vi "Align with Shape.vi"(7 "Margin":cluster{"Horizontal":u32, "Vertical":u32}, 8 "error in (no error)":errorcluster, 9 "Alignment":T1(ring), 10 "Reference Shape":refnum<class "Shape.lvclass">, 11 "Shape in":refnum<class "Shape.lvclass">) -> (0 "error out":errorcluster, 3 "Shape out":refnum<class "Shape.lvclass">)   [LabVIEW 2015, in "LV Image Editor Framework.lvlib" / "Shape.lvclass"]
uses:
  Shape.lvclass
  Shape.lvclass/Shape.ctl
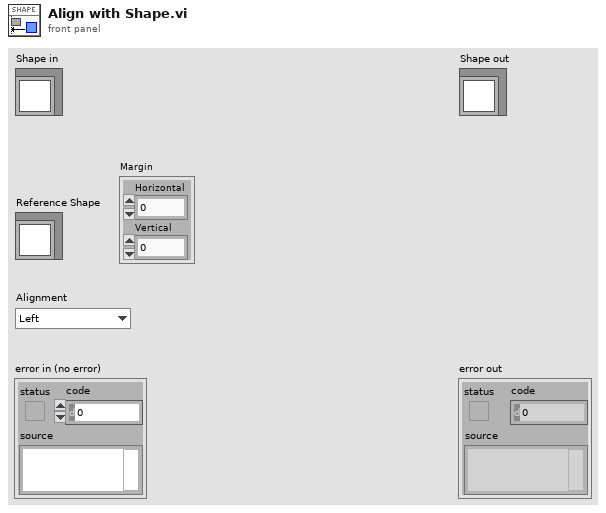
[diagram p1: front panel]
types:
  T1 = enum16{"Left", "Top", "Right", "Bottom", "Centered"}
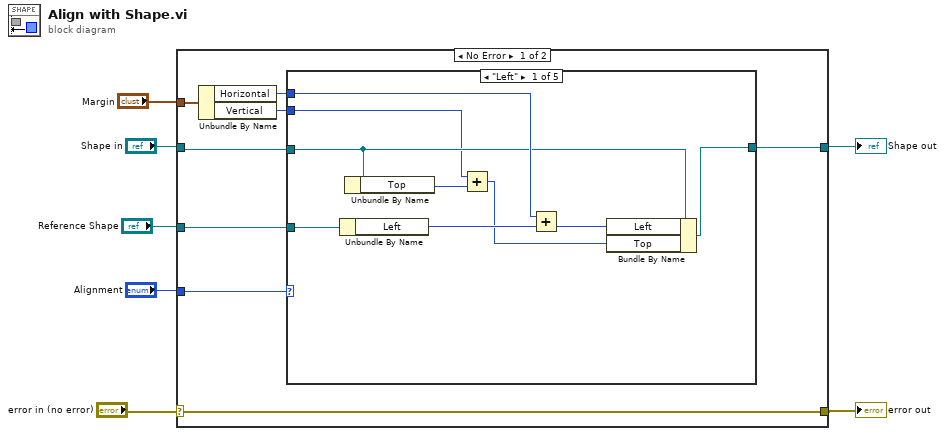
[diagram p0: block diagram]
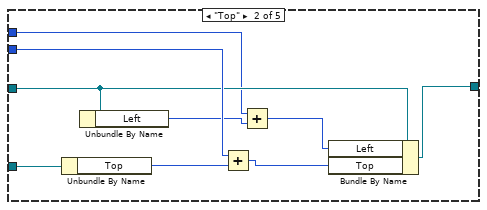
[diagram p2: hidden frame]
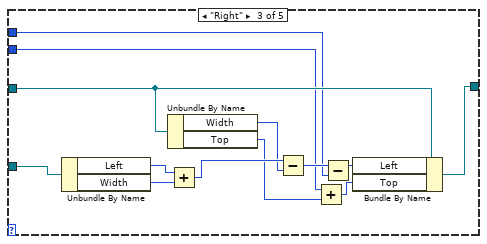
[diagram p3: hidden frame]
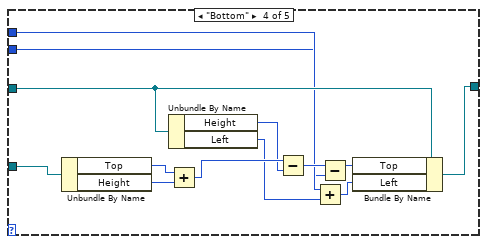
[diagram p4: hidden frame]
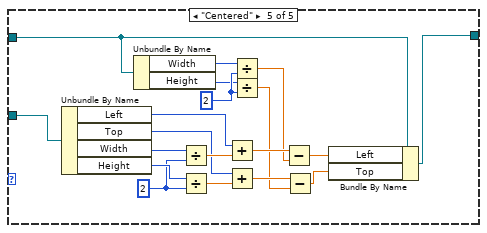
[diagram p5: hidden frame]
diagram:
  n1 = case shown="No Error" "error in (no error)" {
    selector: "error in (no error)" -> [w15 w80]
    tunnel: [w15 w80] -> w6
    tunnel: [w11 w79] -> w2
    tunnel: "Shape in" -> [w13 w79]
    tunnel: "Alignment" -> [w14 _]
    tunnel: "Reference Shape" -> [w12 _]
    tunnel: "Margin" -> [w10 _]
    frame No Error {
      n2 = Unbundle By Name(w10) -> ("Horizontal"=w9:u32, "Vertical"=w8:u32)
      n3 = case shown="\"Left\"" w14 {
        tunnel: w13 -> [w19 w29 w44 w57 w69]
        tunnel: w12 -> [w24 w33 w46 w59 w78]
        tunnel: [w22 w31 w45 w58 w77] -> w11
        tunnel: w9 -> [w20 w26 w35 w51 _]
        tunnel: w8 -> [w17 w30 w37 w48 _]
        frame "Left" {
          n4 = Unbundle By Name(w24) -> ("Left"=w23:i32)
          n5 = Unbundle By Name(w19) -> ("Top"=w18:i32)
          n6 = Add(x=w17, y=w18) -> (x+y=w16:u32)
          n7 = Add(x=w20, y=w23) -> (x+y=w21:u32)
          n8 = Bundle By Name(cluster=w19, "Left"=w21, "Top"=w16) -> (w22:refnum<class "Shape.lvclass">)
        }
        frame "Top" {
          n9 = Unbundle By Name(w33) -> ("Top"=w32:i32)
          n10 = Unbundle By Name(w29) -> ("Left"=w27:i32)
          n11 = Add(x=w30, y=w32) -> (x+y=w28:u32)
          n12 = Add(x=w26, y=w27) -> (x+y=w25:u32)
          n13 = Bundle By Name(cluster=w29, "Left"=w25, "Top"=w28) -> (w31:refnum<class "Shape.lvclass">)
        }
        frame "Right" {
          n14 = Unbundle By Name(w46) -> ("Left"=w43:i32, "Width"=w42:i32)
          n15 = Unbundle By Name(w44) -> ("Width"=w40:i32, "Top"=w34:i32)
          n16 = Add(x=w43, y=w42) -> (x+y=w41:i32)
          n17 = Subtract(x=w41, y=w40) -> (x-y=w39:i32)
          n18 = Add(x=w37, y=w34) -> (x+y=w38:u32)
          n19 = Subtract(x=w39, y=w35) -> (x-y=w36:u32)
          n20 = Bundle By Name(cluster=w44, "Left"=w36, "Top"=w38) -> (w45:refnum<class "Shape.lvclass">)
        }
        frame "Bottom" {
          n21 = Unbundle By Name(w59) -> ("Top"=w56:i32, "Height"=w55:i32)
          n22 = Unbundle By Name(w57) -> ("Height"=w53:i32, "Left"=w47:i32)
          n23 = Add(x=w56, y=w55) -> (x+y=w54:i32)
          n24 = Subtract(x=w54, y=w53) -> (x-y=w52:i32)
          n25 = Add(x=w51, y=w47) -> (x+y=w50:u32)
          n26 = Subtract(x=w52, y=w48) -> (x-y=w49:u32)
          n27 = Bundle By Name(cluster=w57, "Top"=w49, "Left"=w50) -> (w58:refnum<class "Shape.lvclass">)
        }
        frame "Centered" {
          w67 = 2 ("y")
          w74 = 2 ("y")
          n28 = Unbundle By Name(w78) -> ("Left"=w73:i32, "Top"=w71:i32, "Width"=w76:i32, "Height"=w75:i32)
          n29 = Unbundle By Name(w69) -> ("Width"=w68:i32, "Height"=w66:i32)
          n30 = Divide(x=w76, y=w74) -> (x/y=w72:dbl)
          n31 = Divide(x=w75, y=w74) -> (x/y=w70:dbl)
          n32 = Add(x=w73, y=w72) -> (x+y=w65:dbl)
          n33 = Add(x=w71, y=w70) -> (x+y=w63:dbl)
          n34 = Divide(x=w68, y=w67) -> (x/y=w64:dbl)
          n35 = Divide(x=w66, y=w67) -> (x/y=w62:dbl)
          n36 = Subtract(x=w65, y=w64) -> (x-y=w61:dbl)
          n37 = Subtract(x=w63, y=w62) -> (x-y=w60:dbl)
          n38 = Bundle By Name(cluster=w69, "Left"=w61, "Top"=w60) -> (w77:refnum<class "Shape.lvclass">)
        }
      }
    }
    frame Error {
    }
  }
  "error out" <- w6
  "Shape out" <- w2
